vi "ResolveLogosURLMachineAlias.vi"(8 "error in (no error)":errorcluster, 10 "App Refnum":refnum<vi>, 11 "Unresolved URL":string) -> (0 "error out":errorcluster, 3 "Resolved URL":string)   [LabVIEW 2020]
uses:
  <vilib>/Utility/error.llb/whitespace.ctl
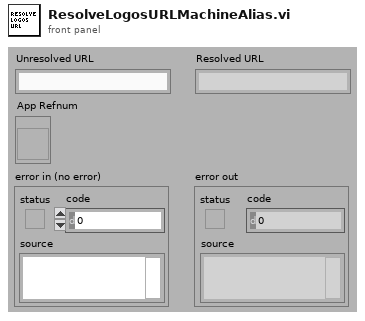
[diagram p1: front panel]
types:
  T1 = typedef "whitespace.ctl" = u16
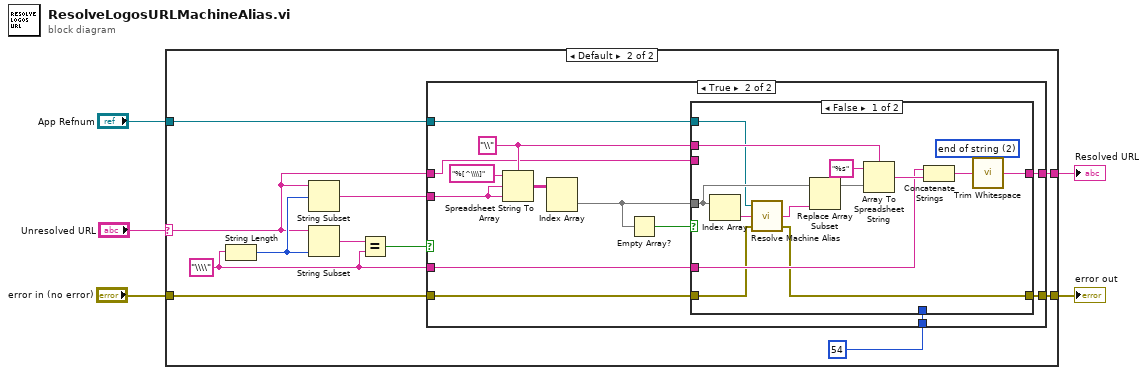
[diagram p0: block diagram]
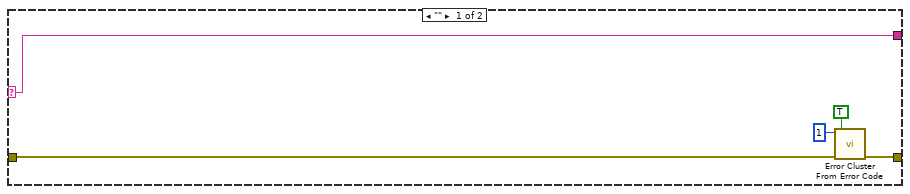
[diagram p2: hidden frame]
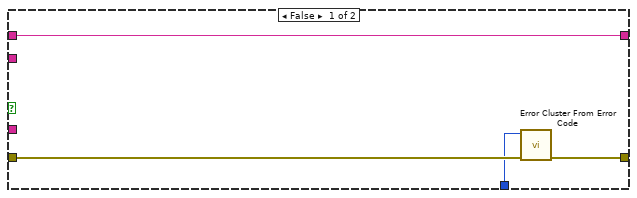
[diagram p3: hidden frame]
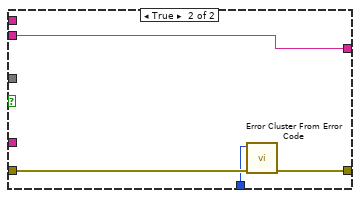
[diagram p4: hidden frame]
diagram:
  n1 = case shown="Default" "Unresolved URL" {
    selector: "Unresolved URL" -> [w10 w11]
    tunnel: [w10 w16] -> w5
    tunnel: "error in (no error)" -> [w8 w15]
    tunnel: [w9 w14] -> w3
    tunnel: "App Refnum" -> [_ w12]
    frame "" {
      n2 = call <vilib>:"Error Cluster From Error Code.vi"("show call chain? (False)"=TRUE, "error in (no error)"=w8, "error code (0)"=1) -> ("error out"=w9:errorcluster)  [unwired: 6 in]
    }
    frame Default {
      w17 = "\\\\" ("format string")
      n3 = String Length(string=w17) -> (length=w19:i32)
      n4 = String Subset(string=w11, offset (0)=w19) -> (substring=w18:string)  [unwired: 1 in]
      n5 = String Subset(string=w11, length (rest)=w19) -> (substring=w21:string)  [unwired: 1 in]
      n6 = Equal?(x=w21, y=w17) -> (x = y?=w20:bool)
      n7 = case shown="True" w20 {
        tunnel: w18 -> [_ w37]
        tunnel: w17 -> [_ w35]
        tunnel: [w25 w34] -> w16
        tunnel: w15 -> [w23 w33]
        tunnel: [w24 w32] -> w14
        tunnel: w11 -> [w25 w30]
        tunnel: 54 ("error code (0)") -> [w22 w27]
        tunnel: w12 -> [_ w26]
        frame False {
          n8 = call <vilib>:"Error Cluster From Error Code.vi"("error in (no error)"=w23, "error code (0)"=w22) -> ("error out"=w24:errorcluster)  [unwired: 7 in]
        }
        frame True {
          w31 = "\\" ("delimiter (Tab)")
          n9 = Spreadsheet String To Array(delimiter (Tab)=w31, format string="%[^\\\\]", spreadsheet string=w37, array type (2D Dbl)=w37) -> (array=w36:string[][])
          n10 = Index Array(array=w36) -> (element=w29:string[])  [unwired: 2 in]
          n11 = Empty Array?(array=w29) -> (empty?=w28:bool)
          n12 = case shown="False" w28 {
            tunnel: w35 -> [w48 _]
            tunnel: [w41 w56] -> w34
            tunnel: w33 -> [w47 w54]
            tunnel: [w46 w55] -> w32
            tunnel: w29 -> [w44 _]
            tunnel: w31 -> [w43 _]
            tunnel: w30 -> [_ w56]
            tunnel: w27 -> [_ w53]
            tunnel: w26 -> [w39 _]
            frame False {
              w40 = T1 2 items=["both", "start of string", "end of string"] ("location (both)")
              n13 = Index Array(array=w44) -> (element=w45:string)  [unwired: 1 in]
              n14 = call <vilib>:"Resolve Machine Alias.vi"("error in"=w47, "Machine Alias"=w45, "App Refnum"=w39) -> ("error out"=w46:errorcluster, "Network Identity"=w52:string)  [unwired: 1 out]
              n15 = Replace Array Subset(array=w44, new element=w52) -> (w51:string[])  [unwired: 1 in]
              n16 = Array To Spreadsheet String(delimiter (Tab)=w43, array=w51, 3:"%s" ("format string")) -> (spreadsheet string=w49:string)
              n17 = Concatenate Strings(w48, w49) -> (w42:string)
              n18 = call <vilib>:"Trim Whitespace.vi"("string"=w42, "location (both)"=w40) -> ("trimmed string"=w41:string)
            }
            frame True {
              n19 = call <vilib>:"Error Cluster From Error Code.vi"("error in (no error)"=w54, "error code (0)"=w53) -> ("error out"=w55:errorcluster)  [unwired: 7 in]
            }
          }
        }
      }
    }
  }
  "error out" <- w3
  "Resolved URL" <- w5
